vi "Add_Street_Name_Hack.vi"(0 "Model Input Position":dbl[](array[numeric])=[0.0, 0.0, 0.0] format="%.2f") -> (6 "Street Names":string)   [LabVIEW 2010]
uses:
  Globals/Constants_global.vi
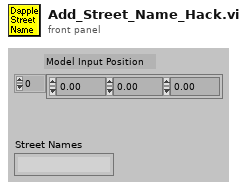
[diagram p1: front panel]
types:
  T1 = enum16{"Load setup from excel file", "Save setup to excel file"}
  T2 = typedef "Exclude_cluster.ctl" = cluster{"Sizes":T3, "Name":string, "Exclude Type":T4}
  T3 = typedef "Box_size.ctl" = cluster{"Max":dbl, "Min":dbl}[]
  T4 = typedef "Exclusion_type.ctl" = enum16{"Exclude completely", "Allow only vertical moves"}
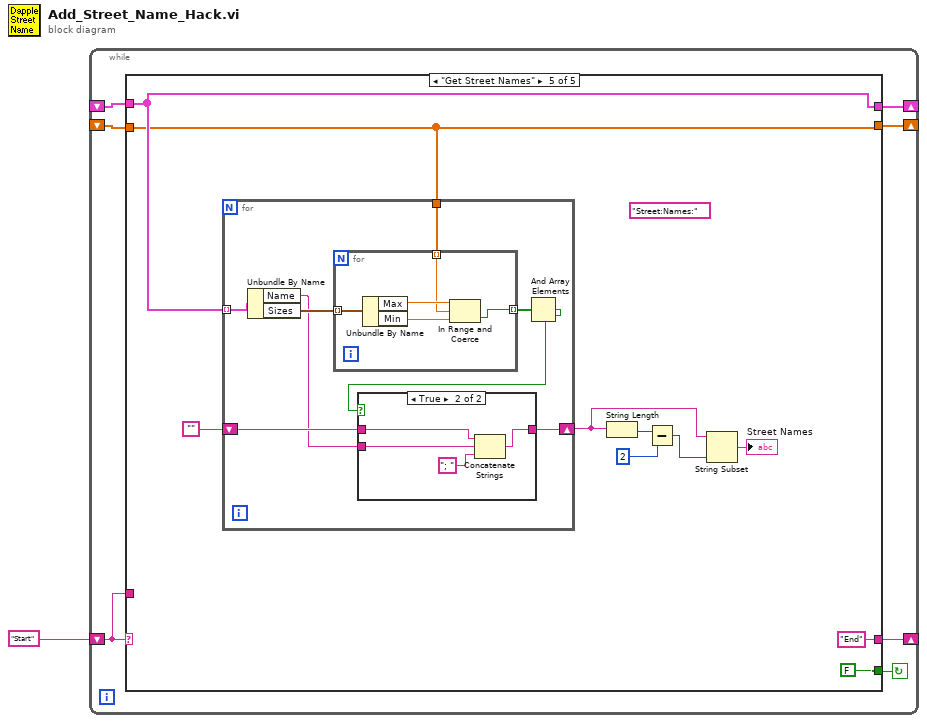
[diagram p0: block diagram]
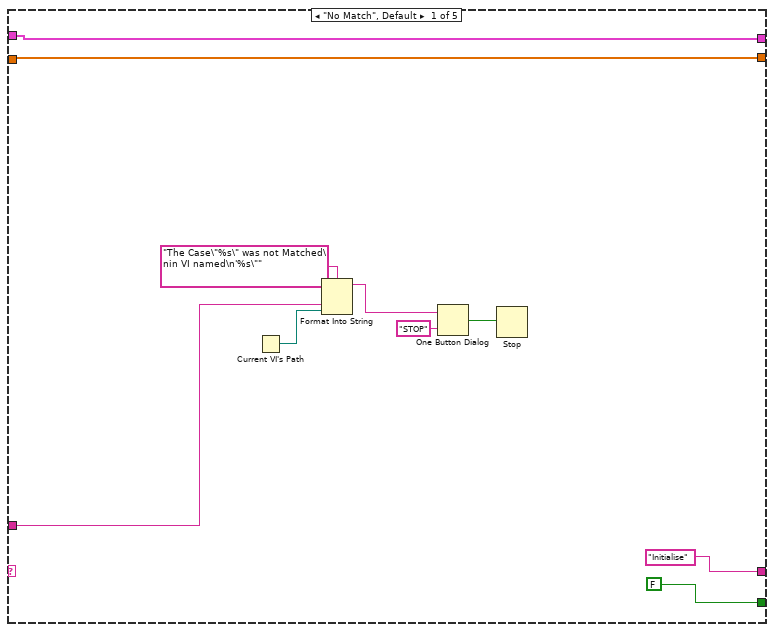
[diagram p2: hidden frame]
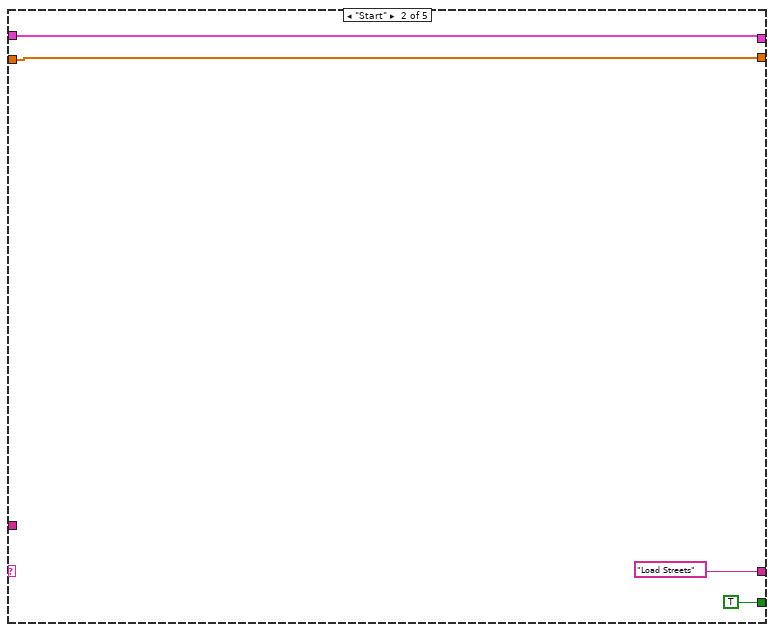
[diagram p3: hidden frame]
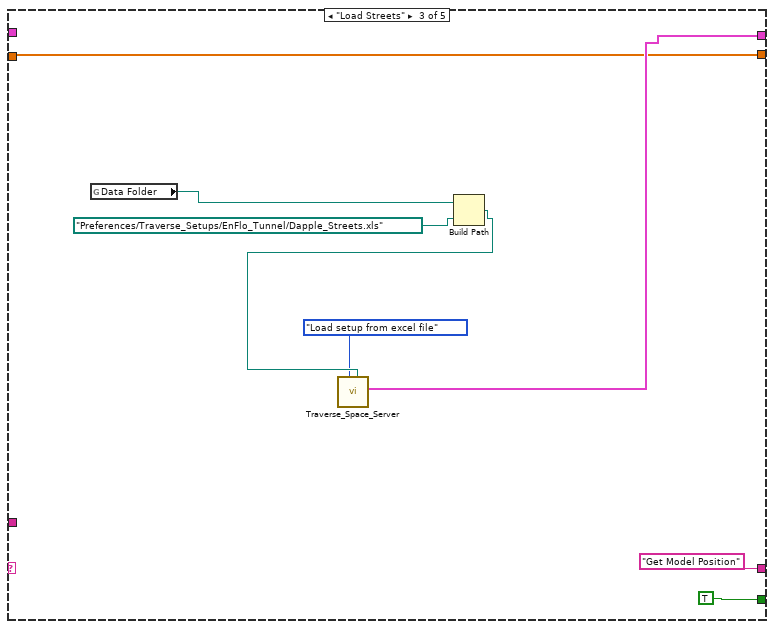
[diagram p4: hidden frame]
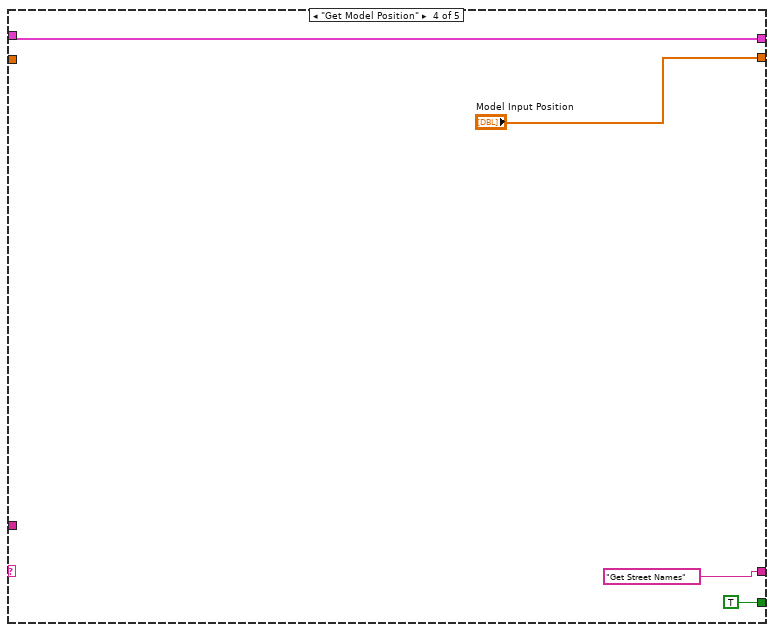
[diagram p5: hidden frame]
diagram:
  n1 = while {
    shift-left: "Start" -> [w6]
    shift-right: [w7] -> _
    shift-right: [w5] -> _
    shift-left: _ -> [w4]
    shift-right: [w3] -> _
    shift-left: _ -> [w2]
    stop <- w8 continue-if-true
    n2 = case shown="\"Get Street Names\"" w6 {
      tunnel: [FALSE TRUE ("Processing last block?") TRUE TRUE ("Processing last block?") FALSE ("Processing last block?")] -> w8
      tunnel: ["Initialise" "Load Streets" "Get Model Position" "Get Street Names" "End"] -> w7
      tunnel: w6 -> [w13 _ _ _ _]
      tunnel: [w10 w21 w24 w34 w37] -> w5
      tunnel: w4 -> [w10 w21 _ w34 w37]
      tunnel: [w9 w20 w23 "Model Input Position" w36] -> w3
      tunnel: w2 -> [w9 w20 w23 _ w36]
      frame "No Match", Default {
        n3 = Current VI's Path() -> (path=w12:path)
        n4 = Format Into String(format string="The Case\"%s\" was not Matched\nin VI named\n'%s\"" ("Format String"), w13, w12) -> (resulting string=w16:string)  [unwired: 2 in, 1 out]
        n5 = One Button Dialog(message=w16, button name ("OK")="STOP") -> (true=w14:bool)
        n6 = Stop(stop? (T)=w14) -> ()
      }
      frame "Start" {
      }
      frame "Load Streets" {
        n7 = global read "Constants_global.vi" "Data Folder"() -> (w28:path)
        n8 = Build Path(base path=w28, name or relative path=path "Preferences/Traverse_Setups/EnFlo_Tunnel/Dapple_Streets.xls") -> (appended path=w26:path)
        n9 = call "Traverse_Space_Server.vi"("Space File"=w26, "Mode"=T1."Load setup from excel file") -> ("Exclude Array Out"=w24:T2[])  [unwired: 5 in, 3 out]
      }
      frame "Get Model Position" {
      }
      frame "Get Street Names" {
        (unwired) "Street:Names:"
        n10 = for {
          tunnel: w37 -> [w52] mode=indexing
          tunnel: w36 -> [w50]
          shift-right: [w46] -> w40
          shift-left: "" -> [w48]
          n11 = Unbundle By Name(w52) -> ("Name"=w47:string, "Sizes"=w51:T3)
          n12 = for {
            tunnel: w51 -> [w62] mode=indexing
            tunnel: w50 -> [w59] mode=indexing
            tunnel: [w58] -> w49 mode=indexing
            n13 = Unbundle By Name(w62) -> ("Max"=w61:dbl, "Min"=w60:dbl)
            n14 = In Range and Coerce(upper limit=w61, x=w59, lower limit=w60) -> (In Range?=w58:bool)  [unwired: 1 out]
          }
          n15 = And Array Elements(Boolean array=w49) -> (logical AND=w45:bool)
          n16 = case shown="True" w45 {
            tunnel: w48 -> [w53 w57]
            tunnel: w47 -> [_ w56]
            tunnel: [w53 w54] -> w46
            frame False {
            }
            frame True {
              n17 = Concatenate Strings(w57, w56, "; " ("string")) -> (w54:string)
            }
          }
        }
        n18 = String Length(string=w40) -> (length=w43:i32)
        n19 = Subtract(x=w43, y=2) -> (x-y=w41:i32)
        n20 = String Subset(string=w40, length (rest)=w41) -> (substring=→"Street Names":string)  [unwired: 1 in]
      }
    }
  }
